vi "RT_Main.vi"() -> ()   [LabVIEW 2016]
uses:
  Application Control/FSM States.ctl
  RTLSDR Control/RTLSDR Global Variables.vi
  <vilib>/Utility/SystemLogging/NI_SystemLogging.lvlib
  <vilib>/nisyscfg/nisyscfg.lvlib
panel:
  out "error IO":errorcluster
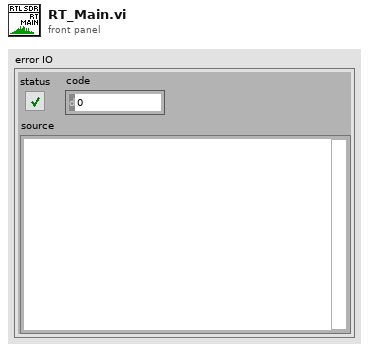
[diagram p1: front panel]
types:
  T1 = typedef "FSM States.ctl" = enum16{"Initialise", "Logging", "Close"}
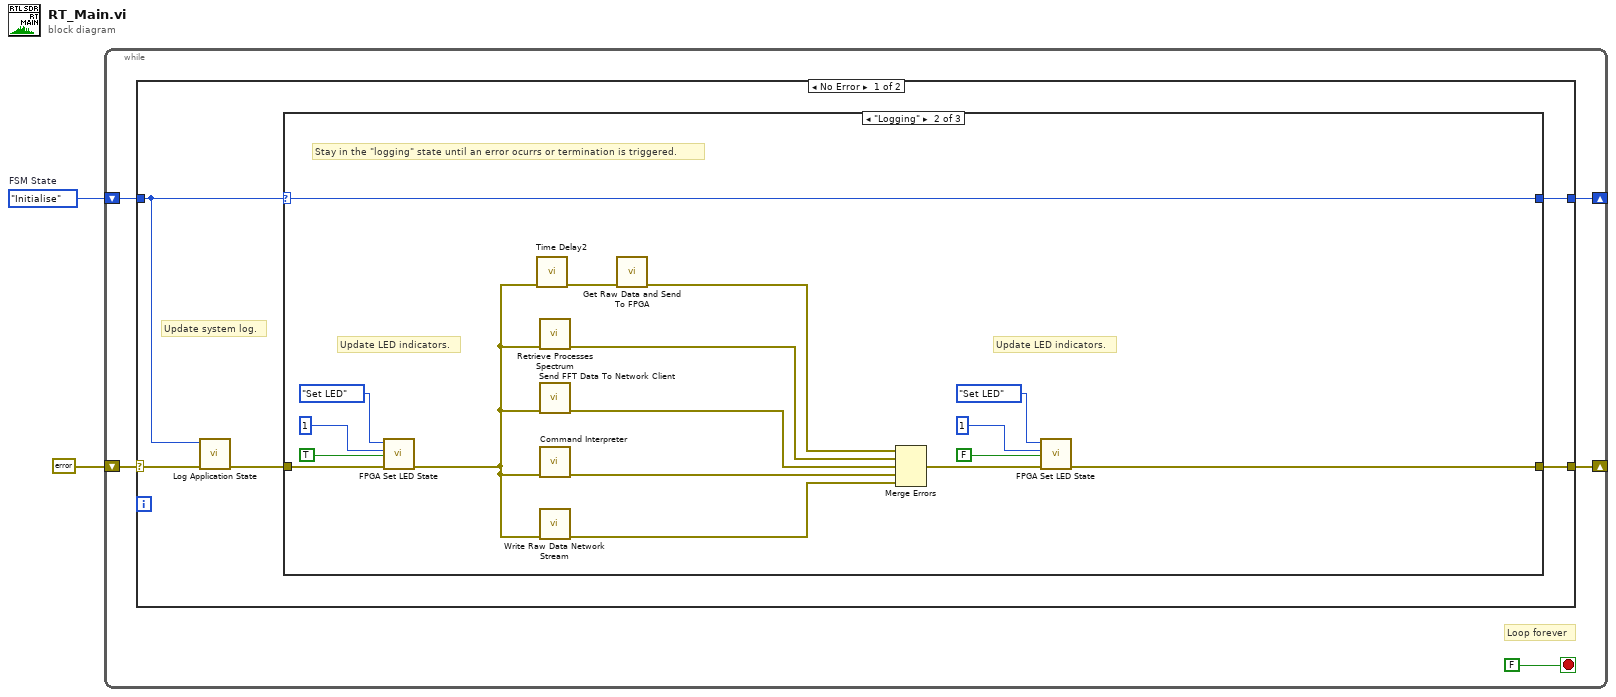
[diagram p0: block diagram]
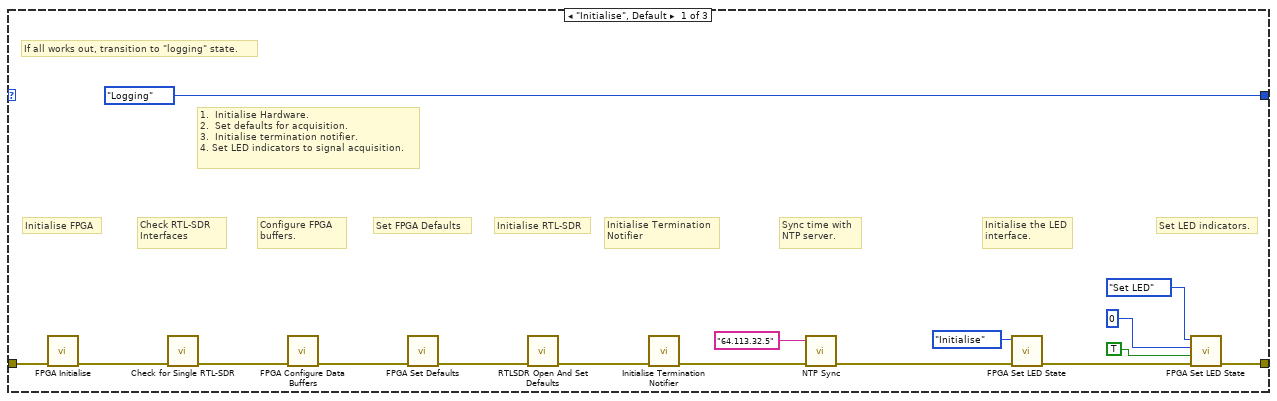
[diagram p2: hidden frame]
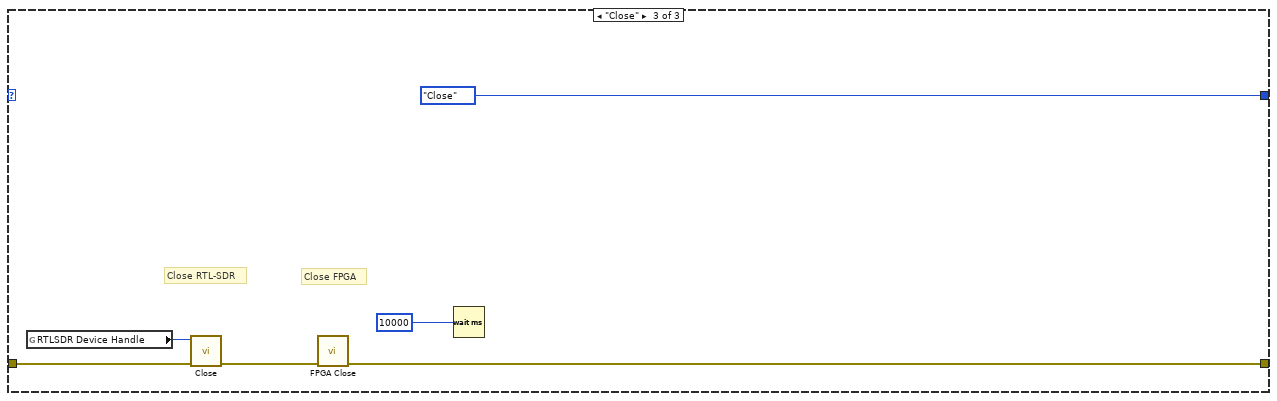
[diagram p3: hidden frame]
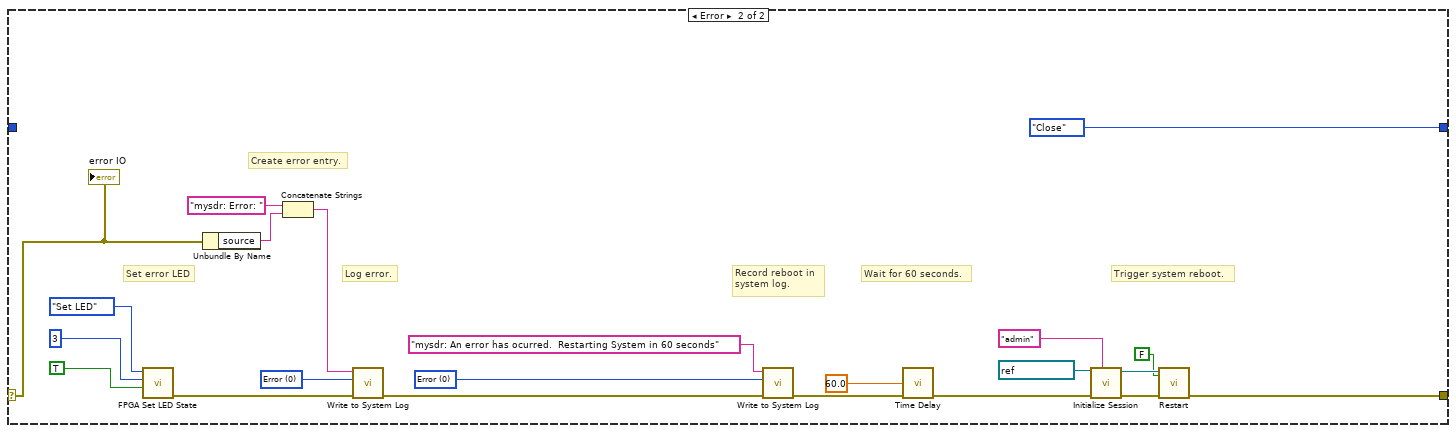
[diagram p4: hidden frame]
diagram:
  w2 = FSM_States."Initialise"  # FSM State
  n1 = while {
    shift-right: [w6] -> _
    shift-left: errorcluster {"status"=FALSE, "code"=0, "source"=""} ("error out") -> [w4]
    shift-right: [w5] -> _
    shift-left: w2 -> [w7]
    stop <- FALSE stop-if-true
    # "Loop forever"
    n2 = case shown="No Error" w4 {
      selector: w4 -> [w9 w52]
      tunnel: w7 -> [w10 _]
      tunnel: [w12 w64] -> w6
      tunnel: [w11 FSM_States."Close"] -> w5
      frame No Error {
        # "Update system log."
        n3 = call "Log Application State.vi"("error in (no error)"=w9, "FSM State"=w10) -> ("error out"=w8:errorcluster)  [unwired: 9 in]
        n4 = case shown="\"Logging\"" w10 {
          selector: w10 -> [_ w41 _]
          tunnel: w8 -> [w26 w40 w50]
          tunnel: [w16 w32 w49] -> w12
          tunnel: [FSM_States."Logging" w41 FSM_States."Close"] -> w11
          frame "Initialise", Default {
            # "Sync time with\nNTP server."
            # "If all works out, transition to \"logging\" state."
            # "1.  Initialise Hardware.\n2.  Set defaults for acquisition.\n3.  Initialise termination notifier.\n4. Set LED indicators to signal acquisition."
            # "Set LED indicators."
            # "Initialise the LED\ninterface."
            # "Initialise Termination\nNotifier"
            # "Initialise RTL-SDR"
            # "Set FPGA Defaults"
            # "Configure FPGA\nbuffers."
            # "Check RTL-SDR \nInterfaces"
            # "Initialise FPGA"
            n5 = call "FPGA Initialise.vi"("error in (no error)"=w26) -> ("error out"=w25:errorcluster)  [unwired: 10 in]
            n6 = call "Check for Single RTL-SDR.vi"("error in (no error)"=w25) -> ("error out"=w24:errorcluster)  [unwired: 10 in]
            n7 = call "FPGA Configure Data Buffers.vi"("error in (no error)"=w24) -> ("error out"=w27:errorcluster)  [unwired: 10 in]
            n8 = call "FPGA Set Defaults.vi"("error in (no error)"=w27) -> ("error out"=w28:errorcluster)  [unwired: 10 in]
            n9 = call "RTLSDR Open And Set Defaults.vi"("error in (no error)"=w28) -> ("error out"=w17:errorcluster)  [unwired: 10 in]
            n10 = call "Initialise Termination Notifier.vi"("error in (no error)"=w17) -> ("error out"=w15:errorcluster)  [unwired: 10 in]
            n11 = call "NTP Sync.vi"("error in (no error)"=w15, "Time Server IP"="64.113.32.5") -> ("error out"=w14:errorcluster)  [unwired: 7 in, 2 out]
            n12 = call "FPGA Set LED State.vi"("error in (no error)"=w14, "Command"=enum16{"Set LED", "Initialise"}."Initialise") -> ("error out"=w21:errorcluster)  [unwired: 9 in]
            n13 = call "FPGA Set LED State.vi"("error in (no error)"=w21, "State"=TRUE, "LED"=u8 0, "Command"=enum16{"Set LED", "Initialise"}."Set LED") -> ("error out"=w16:errorcluster)  [unwired: 7 in]
          }
          frame "Logging" {
            # "Stay in the \"logging\" state until an error ocurrs or termination is triggered."
            # "Update LED indicators."
            # "Update LED indicators."
            n14 = call "FPGA Set LED State.vi"("error in (no error)"=w40, "State"=TRUE, "LED"=u8 1, "Command"=enum16{"Set LED", "Initialise"}."Set LED") -> ("error out"=w30:errorcluster)  [unwired: 7 in]
            n15 = call "Time Delay2"("error in (no error)"=w30) -> ("error out"=w29:errorcluster)  [unwired: 10 in]
            n16 = call "Retrieve Processes Spectrum.vi"("error in (no error)"=w30) -> ("error out"=w44:errorcluster)  [unwired: 10 in]
            n17 = call "Send FFT Data To Network Client.vi"("error in (no error)"=w30) -> ("error out"=w42:errorcluster)  [unwired: 10 in]
            n18 = call "Command Interpreter.vi"("error in (no error)"=w30) -> ("error out"=w43:errorcluster)  [unwired: 10 in]
            n19 = call "Write Raw Data Network Stream.vi"("error in (no error)"=w30) -> ("error out"=w31:errorcluster)  [unwired: 10 in]
            n20 = call "Get Raw Data and Send To FPGA.vi"("error in (no error)"=w29) -> ("error out"=w45:errorcluster)  [unwired: 10 in]
            n21 = Merge Errors(w45, w44, w42, w43, w31) -> (w33:errorcluster)
            n22 = call "FPGA Set LED State.vi"("error in (no error)"=w33, "State"=FALSE, "LED"=u8 1, "Command"=enum16{"Set LED", "Initialise"}."Set LED") -> ("error out"=w32:errorcluster)  [unwired: 7 in]
          }
          frame "Close" {
            # "Close FPGA"
            # "Close RTL-SDR"
            n23 = global read "RTLSDR Global Variables.vi" "RTLSDR Device Handle"() -> (w48:u64)
            n24 = call "Close.vi"("error in (no error)"=w50, "DeviceRefnum"=w48) -> ("error out"=w51:errorcluster)  [unwired: 8 in, 1 out]
            n25 = call "FPGA Close.vi"("error in (no error)"=w51) -> ("error out"=w49:errorcluster)  [unwired: 10 in]
            n26 = Wait (ms)(milliseconds to wait=u32 10000) -> ()  [unwired: 1 out]
          }
        }
      }
      frame Error {
        w70 = 0 items=["Error", "Warning", "Informational"] ("severity")
        w73 = 0 items=["Error", "Warning", "Informational"] ("severity")
        # "Create error entry."
        # "Set error LED"
        # "Log error."
        # "Trigger system reboot."
        # "Wait for 60 seconds."
        # "Record reboot in\nsystem log."
        n27 = call "FPGA Set LED State.vi"("State"=TRUE, "LED"=u8 3, "Command"=enum16{"Set LED", "Initialise"}."Set LED") -> ("error out"=w53:errorcluster)  [unwired: 8 in]
        n28 = Unbundle By Name(w52) -> ("source"=w58:string)
        n29 = Concatenate Strings("mysdr: Error: " ("string"), w58) -> (w57:string)
        n30 = call <vilib>:"Write to System Log.vi"("error in (no error)"=w53, "severity"=w73, "message"=w57) -> ("error out"=w71:errorcluster)  [unwired: 8 in]
        n31 = call <vilib>:"Write to System Log.vi"("error in (no error)"=w71, "severity"=w70, "message"="mysdr: An error has ocurred.  Restarting System in 60 seconds") -> ("error out"=w63:errorcluster)  [unwired: 8 in]
        n32 = call "Time Delay"("error in (no error)"=w63, "Delay Time (s)"=60.0) -> ("error out"=w62:errorcluster)  [unwired: 9 in]
        n33 = call <vilib>:"Initialize Session.vi"("User Name"="admin", "error in (no error)"=w62, "Target (localhost)"=refnum<k21> "localhost") -> ("error out"=w66:errorcluster, "Session out"=w68:refnum<k21>)  [unwired: 7 in]
        n34 = call <vilib>:"Restart.vi"("Wait Until Complete (T)"=FALSE, "error in (no error)"=w66, "Session in"=w68) -> ("error out"=w64:errorcluster)  [unwired: 6 in, 2 out]
        "error IO" <- w52
      }
    }
  }
